vi "ParseSaxStatus.vi"(1 "Status Code In":u32) -> (0 "Status Flags":i8[](array[numeric]))   [LabVIEW 2014]
panel:
  out "Code Shift":i8[](array[numeric])
  out "Code Mask":i8[](array[numeric])
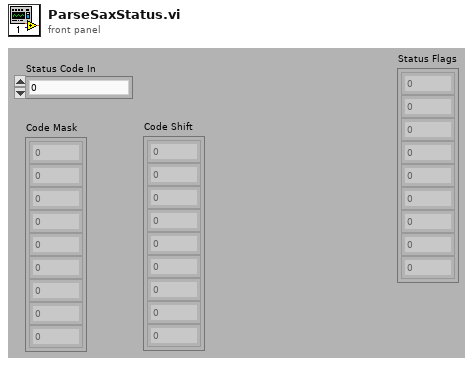
[diagram p1: front panel]
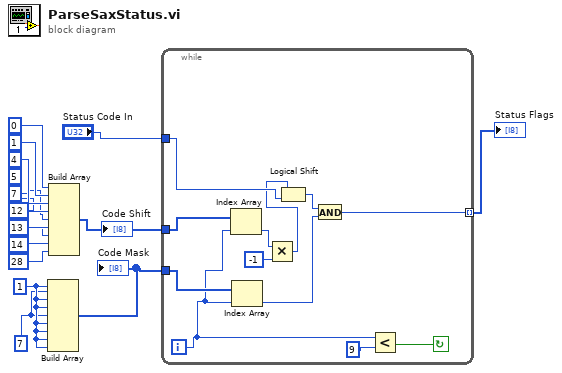
[diagram p0: block diagram]
diagram:
  w12 = 7
  w13 = 1
  n1 = Build Array(w13, w12, w13, w13, w12, w13, w13, w13, w13) -> (w11:i32[])
  "Code Mask" <- w11
  n2 = Build Array(0, 1, 4, 5, 7, 12, 13, 14, 28) -> (w1:i32[])
  "Code Shift" <- w1
  n3 = while {
    tunnel: w11 -> [w25]
    tunnel: w1 -> [w24]
    tunnel: "Status Code In" -> [w17]
    tunnel: [w19] -> w14 mode=indexing
    i -> [w18]
    stop <- w26 continue-if-true
    n4 = Index Array(array=w24, index=w18) -> (element=w22:i32)
    n5 = Index Array(array=w25, index=w18) -> (element=w20:i32)
    n6 = Multiply(x=w22, y=-1) -> (x*y=w16:i32)
    n7 = Logical Shift(y=w16, x=w17) -> (x << y=w21:u32)
    n8 = And(x=w21, y=w20) -> (x .and. y?=w19:u32)
    n9 = Less?(x=w18, y=9) -> (x < y?=w26:bool)
  }
  "Status Flags" <- w14
